vi "select_seat_comfirm.vi"(1 "choose index":i32) -> (0 "Boolean":bool=TRUE)   [LabVIEW 2014]
panel:
  out "concatenated string":string
  in  "Cluster 2":cluster{"OK Button":bool, "Cancel Button":bool}
  out "column":i32
  out "row":i32
  # "The seat you choose is:"
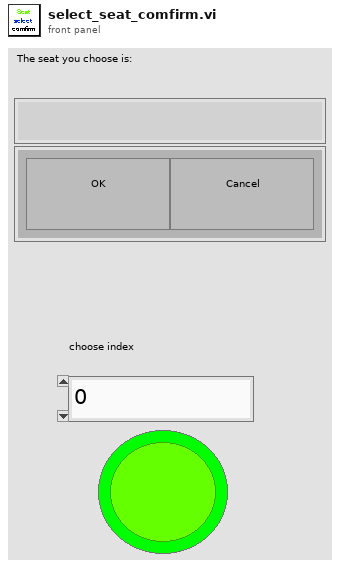
[diagram p1: front panel]
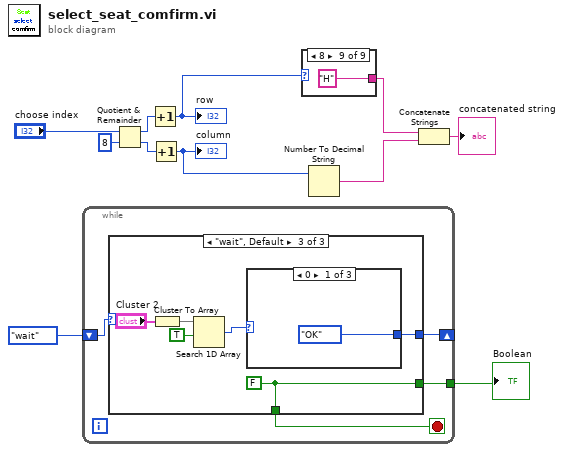
[diagram p0: block diagram]
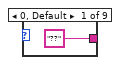
[diagram p2: hidden frame]
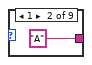
[diagram p3: hidden frame]
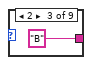
[diagram p4: hidden frame]
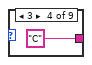
[diagram p5: hidden frame]
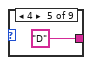
[diagram p6: hidden frame]
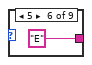
[diagram p7: hidden frame]
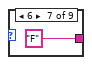
[diagram p8: hidden frame]
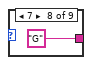
[diagram p9: hidden frame]
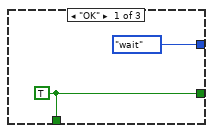
[diagram p10: hidden frame]
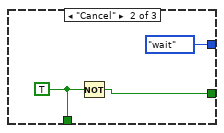
[diagram p11: hidden frame]
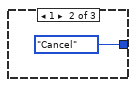
[diagram p12: hidden frame]
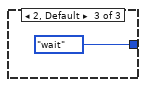
[diagram p13: hidden frame]
diagram:
  n1 = while {
    shift-right: [w14] -> _
    shift-left: enum16{"OK", "Cancel", "wait"}."wait" -> [w15]
    tunnel: [w12] -> w6
    stop <- w13 stop-if-true
    n2 = case shown="\"wait\", Default" w15 {
      tunnel: [enum16{"OK", "Cancel", "wait"}."wait" enum16{"OK", "Cancel", "wait"}."wait" w22] -> w14
      tunnel: [w16 w19 w21] -> w13
      tunnel: [w16 w18 w21] -> w12
      frame "OK" {
        w16 = TRUE
      }
      frame "Cancel" {
        w19 = TRUE
        n3 = Not(x=w19) -> (.not. x?=w18:bool)
      }
      frame "wait", Default {
        w21 = FALSE
        n4 = Cluster To Array(cluster="Cluster 2") -> (array=w25:bool[])
        n5 = Search 1D Array(1D array=w25, element=TRUE) -> (index of element=w23:i32)  [unwired: 1 in]
        n6 = case shown="0" w23 {
          tunnel: [enum16{"OK", "Cancel", "wait"}."OK" enum16{"OK", "Cancel", "wait"}."Cancel" enum16{"OK", "Cancel", "wait"}."wait"] -> w22
          frame 0 {
          }
          frame 1 {
          }
          frame 2, Default {
          }
        }
      }
    }
  }
  "Boolean" <- w6
  n7 = Quotient & Remainder(x="choose index", y=8) -> (x-y*floor(x/y)=w10:i32, floor(x/y)=w9:i32)
  n8 = Increment(x=w10) -> (x+1=w5:i32)
  "row" <- w5
  n9 = Increment(x=w9) -> (x+1=w4:i32)
  "column" <- w4
  n10 = case shown="8" w5 {
    tunnel: ["??" "A" "B" "C" "D" "E" "F" "G" "H"] -> w3
    frame 0, Default {
    }
    frame 1 {
    }
    frame 2 {
    }
    frame 3 {
    }
    frame 4 {
    }
    frame 5 {
    }
    frame 6 {
    }
    frame 7 {
    }
    frame 8 {
    }
  }
  n11 = Number To Decimal String(number=w4) -> (decimal integer string=w2:string)  [unwired: 1 in]
  n12 = Concatenate Strings(w3, w2) -> (→"concatenated string":string)
